vi "Status LED.vi"() -> ()   [LabVIEW 2020, in "CTI-Visa-Scratchpad.lvlib"]
uses:
  CTI-Visa-Scratchpad.lvlib
  CTI-Visa/CTI-Visa.lvlib
  CTI-Visa/Status Source.ctl
panel:
  in  "User Status":bool
  in  "Speed":i32(slide)=101 scale=1000.0..1.0
  in  "stop":bool
  in  "Port":refnum<visa-resource-name>="COM3"
  out "Current Source":T1
  out "ADC":u16(graph)
  in  "User Source":bool
  in  "Comms Source":bool
  # "Set Source:"
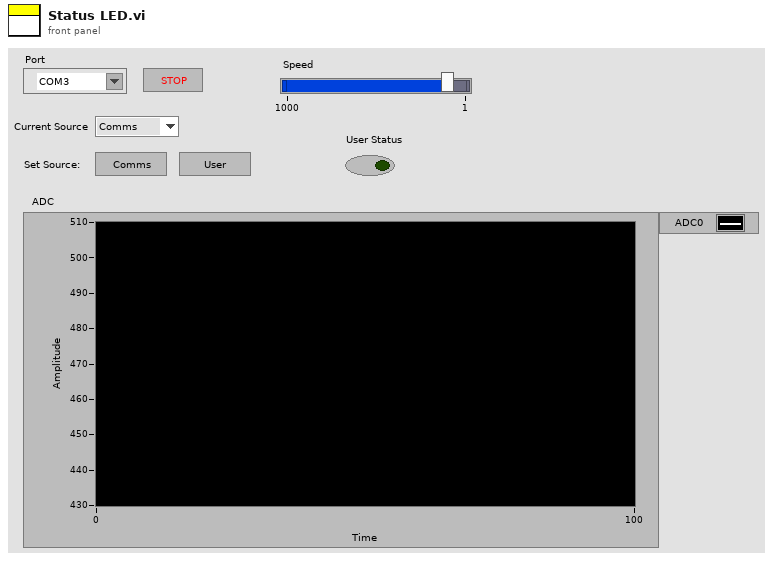
[diagram p1: front panel]
types:
  T1 = typedef "CTI-Visa.lvlib/Status Source.ctl" = enum16{"Comms", "User"}
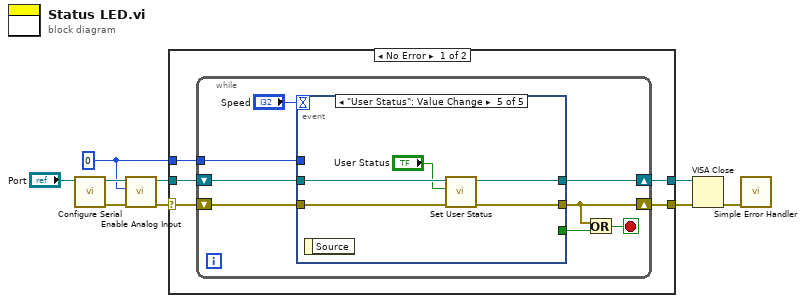
[diagram p0: block diagram]
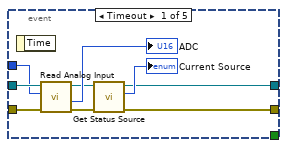
[diagram p2: hidden frame]
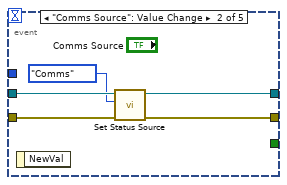
[diagram p3: hidden frame]
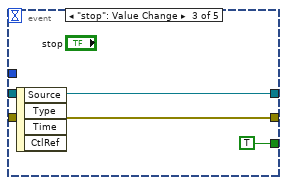
[diagram p4: hidden frame]
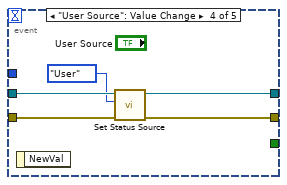
[diagram p5: hidden frame]
diagram:
  w4 = 0 ("Channel")
  n1 = call "Configure Serial.vi"("VISA resource name in"="Port") -> ("error out"=w7:errorcluster, "VISA resource name"=w8:refnum<visa-resource-name>)  [unwired: 9 in]
  n2 = call "Enable Analog Input.vi"("error in (no error)"=w7, "Channel"=w4, "VISA resource name in"=w8) -> ("error out"=w6:errorcluster, "VISA resource name"=w5:refnum<visa-resource-name>)  [unwired: 7 in]
  n3 = case shown="No Error" w6 {
    selector: w6 -> [w13 w50]
    tunnel: w5 -> [w14 w51]
    tunnel: w4 -> [w12 _]
    tunnel: [w11 w51] -> w2
    tunnel: [w10 w50] -> w1
    frame No Error {
      n4 = while {
        shift-right: [w17] -> w10
        shift-left: w13 -> [w20]
        shift-right: [w18] -> w11
        shift-left: w14 -> [w21]
        tunnel: w12 -> [w19]
        stop <- w16 stop-if-true
        n5 = event shown="[4] \"User Status\": Value Change" {
          selector: _ -> [_ _ _ _ _]
          dyn-events: _ -> [_ _ _ _ _]
          timeout: "Speed" -> [_ _ _ _ _]
          tunnel: w21 -> [w31 w36 w39 w44 w49]
          tunnel: w20 -> [w30 w35 w38 w43 w48]
          tunnel: w19 -> [w29 _ _ _ _]
          tunnel: [w24 w33 w39 w41 w46] -> w18
          tunnel: [w23 w32 w38 w40 w47] -> w17
          tunnel: [_ _ TRUE _ _] -> w15
          event Timeout {
            n6 = event-data() -> ()  [unwired: 1 in, 1 out]
            n7 = call "Read Analog Input.vi"("error in (no error)"=w30, "Channel"=w29, "VISA resource name in"=w31) -> ("error out"=w26:errorcluster, "Value"=→"ADC":u16, "VISA resource name"=w27:refnum<visa-resource-name>)  [unwired: 6 in]
            n8 = call "Get Status Source.vi"("error in (no error)"=w26, "VISA resource name in"=w27) -> ("error out"=w23:errorcluster, "Status Source"=→"Current Source":T1, "VISA resource name"=w24:refnum<visa-resource-name>)  [unwired: 7 in]
          }
          event "Comms Source": Value Change {
            n9 = event-data() -> ()  [unwired: 1 in, 1 out]
            n10 = call "Set Status Source.vi"("error in (no error)"=w35, "Status Source"=Status_Source."Comms", "VISA resource name in"=w36) -> ("error out"=w32:errorcluster, "VISA resource name"=w33:refnum<visa-resource-name>)  [unwired: 7 in]
          }
          event "stop": Value Change {
            n11 = event-data() -> ()  [unwired: 1 in, 4 out]
          }
          event "User Source": Value Change {
            n12 = event-data() -> ()  [unwired: 1 in, 1 out]
            n13 = call "Set Status Source.vi"("error in (no error)"=w43, "Status Source"=Status_Source."User", "VISA resource name in"=w44) -> ("error out"=w40:errorcluster, "VISA resource name"=w41:refnum<visa-resource-name>)  [unwired: 7 in]
          }
          event "User Status": Value Change {
            n14 = event-data() -> ()  [unwired: 1 in, 1 out]
            n15 = call "Set User Status.vi"("error in (no error)"=w48, "Value"="User Status", "VISA resource name in"=w49) -> ("error out"=w47:errorcluster, "VISA resource name"=w46:refnum<visa-resource-name>)  [unwired: 7 in]
          }
        }
        n16 = Or(x=w17, y=w15) -> (x .or. y?=w16:bool)
      }
    }
    frame Error {
    }
  }
  n17 = VISA Close(VISA resource name=w2, error in (no error)=w1) -> (error out=w3:errorcluster)
  n18 = call <vilib>:"Simple Error Handler.vi"("error in (no error)"=w3) -> ()  [unwired: 4 in, 5 out]
